vi "Append to Text File.vi"(8 "Error In":errorcluster, 9 "Max Size in Bytes (-1)":i64=-1, 10 "Text":string, 11 "Path (Dialog)":path) -> (0 "Error Out":errorcluster, 3 "Path Out":path)   [LabVIEW 2015, in "Endigit.lvlib"]
doc: "Append \"Text\" to the file at \"Path\". Note: This VI opens and closes the specified file each time it is called.\n\nAuthored by Robert C. Mortensen\nrobert@endigit.com\n\nCopyright (c) 2012, Endigit, Inc.\n\nAll rights reserved.\n\nRedistribution and use in source and binary forms, with or without modification, are permitted provided that the following conditions are met:\n\n * Redistributions of source code must retain the above copyright notice, this list of conditions and the following disclaimer.\n * Redistributions in binary form must reproduce the above copyright notice, this list of conditions and the following disclaimer in the documentation and/or other materials provided with the distribution.\n * Neither the name of Moore Good Ideas, Inc. nor the names of its contributors may be used to endorse or promote products derived from this software without specific prior written permission.\n\nTHIS SOFTWARE IS PROVIDED BY THE COPYRIGHT HOLDERS AND CONTRIBUTORS \"AS IS\" AND ANY EXPRESS OR IMPLIED WARRANTIES, INCLUDING, BUT NOT LIMITED TO, THE IMPLIED WARRANTIES OF MERCHANTABILITY AND FITNESS FOR A PARTICULAR PURPOSE ARE DISCLAIMED. IN NO EVENT SHALL THE COPYRIGHT OWNER OR CONTRIBUTORS BE LIABLE FOR ANY DIRECT, INDIRECT, INCIDENTAL, SPECIAL, EXEMPLARY, OR CONSEQUENTIAL DAMAGES (INCLUDING, BUT NOT LIMITED TO, PROCUREMENT OF SUBSTITUTE GOODS OR SERVICES; LOSS OF USE, DATA, OR PROFITS; OR BUSINESS INTERRUPTION) HOWEVER CAUSED AND ON ANY THEORY OF LIABILITY, WHETHER IN CONTRACT, STRICT LIABILITY, OR TORT (INCLUDING NEGLIGENCE OR OTHERWISE) ARISING IN ANY WAY OUT OF THE USE OF THIS SOFTWARE, EVEN IF ADVISED OF THE POSSIBILITY OF SUCH DAMAGE."
uses:
  Endigit.lvlib
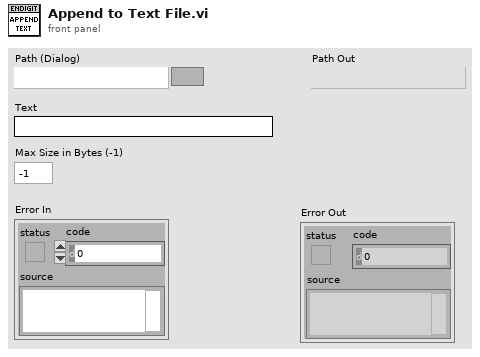
[diagram p1: front panel]
types:
  T1 = enum16{"open", "replace", "create", "open or create", "replace or create", "replace or create with confirmation"}
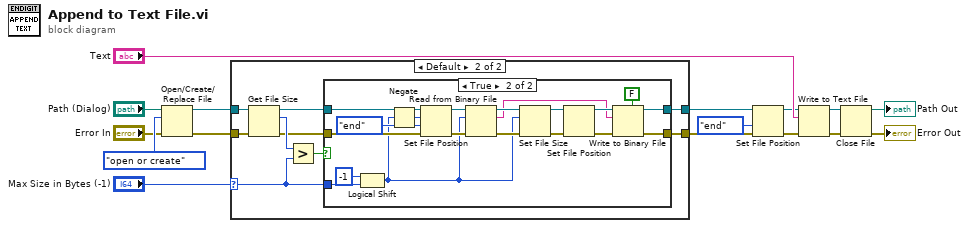
[diagram p0: block diagram]
diagram:
  n1 = Open/Create/Replace File(file path (use dialog)="Path (Dialog)", error in="Error In", operation (0:open)=T1."open or create") -> (refnum out=w12:refnum<file>, error out=w11:errorcluster)  [unwired: 3 in, 1 out]
  n2 = case shown="Default" "Max Size in Bytes (-1)" {
    selector: "Max Size in Bytes (-1)" -> [_ w19]
    tunnel: w12 -> [w18 w27]
    tunnel: w11 -> [w17 w26]
    tunnel: [w18 w23] -> w10
    tunnel: [w17 w21] -> w9
    frame -1 {
    }
    frame Default {
      n3 = Get File Size(file=w27, error in=w26) -> (refnum out=w22:refnum<file>, size (in bytes)=w25:i64, 0:w20:errorcluster)
      n4 = Greater?(x=w25, y=w19) -> (0:w24:bool)
      n5 = case shown="True" w24 {
        tunnel: [w29 w32] -> w23
        tunnel: w22 -> [w29 w46]
        tunnel: [w28 w33] -> w21
        tunnel: w20 -> [w28 w45]
        tunnel: w19 -> [_ w48]
        frame False {
        }
        frame True {
          n6 = Logical Shift(y=i16 -1, x=w48) -> (x << y=w38:i64)
          n7 = Negate(x=w38) -> (-x=w41:i64)
          n8 = Set File Position(offset (in bytes) (0)=w41, refnum=w46, from (0:start)=enum16{"start", "end", "current"}."end", error in=w45) -> (refnum out=w44:refnum<file>, error out=w43:errorcluster)
          n9 = Read from Binary File(8:w43, 10:w38, 11:w44) -> (0:w39:errorcluster, 2:w31:string, 3:w40:refnum<file>)  [unwired: 3 in, 1 out]
          n10 = Set File Size(4:w39, 6:w38, 7:w40) -> (0:w36:errorcluster, 3:w37:refnum<file>)
          n11 = Set File Position(refnum=w37, error in=w36) -> (refnum out=w34:refnum<file>, error out=w35:errorcluster)  [unwired: 2 in]
          n12 = Write to Binary File(file (use dialog)=w34, data=w31, error in=w35, 5:FALSE ("prepend array or string size? (T)")) -> (refnum out=w32:refnum<file>, error out=w33:errorcluster)  [unwired: 2 in, 1 out]
        }
      }
    }
  }
  n13 = Set File Position(refnum=w10, from (0:start)=enum16{"start", "end", "current"}."end", error in=w9) -> (refnum out=w7:refnum<file>, error out=w8:errorcluster)  [unwired: 1 in]
  n14 = Write to Text File(file (use dialog)=w7, text="Text", error in=w8) -> (refnum out=w5:refnum<file>, error out=w6:errorcluster)  [unwired: 2 out]
  n15 = Close File(refnum=w5, error in=w6) -> (path=→"Path Out":path, error out=→"Error Out":errorcluster)
